vi "HEWH RLT Write Channels.vi"(8 "Error In":errorcluster, 11 "Panel Input":T1[][](array[typedef])) -> (0 "Error Out":errorcluster, 3 "Write Array":string[][](array[string]))   [LabVIEW 2016]
uses:
  Type Definitions/HEWH Channel Label RLT.ctl
  Custom Instrument Control/MW100/Type Definitions/Station ID Selector.ctl
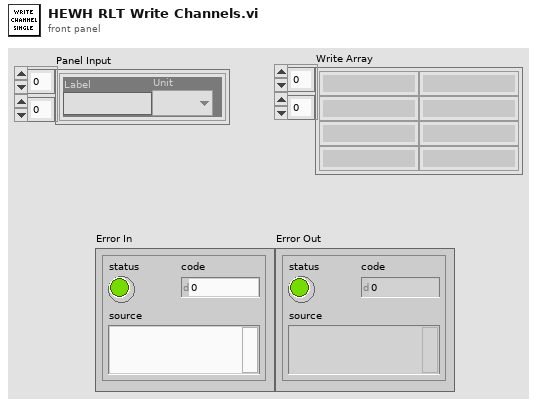
[diagram p1: front panel]
types:
  T1 = typedef "HEWH Channel Label RLT.ctl" = cluster{"Label":string, "Unit":T2}
  T2 = typedef "Station ID Selector.ctl" = enum16{"", "A", "B", "C", "D", "Global"}
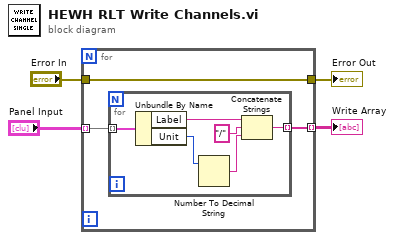
[diagram p0: block diagram]
diagram:
  n1 = for {
    tunnel: "Panel Input" -> [w7] mode=indexing
    tunnel: [w6] -> w4 mode=indexing
    tunnel: "Error In" -> [w5]
    tunnel: [w5] -> w1
    n2 = for {
      tunnel: w7 -> [w13] mode=indexing
      tunnel: [w8] -> w6 mode=indexing
      n3 = Unbundle By Name(w13) -> ("Label"=w11:string, "Unit"=w12:T2)
      n4 = Number To Decimal String(number=w12) -> (decimal integer string=w9:string)  [unwired: 1 in]
      n5 = Concatenate Strings(w11, "/" ("string"), w9) -> (w8:string)
    }
  }
  "Write Array" <- w4
  "Error Out" <- w1
